vi "读电表参数.vi"(4 "脉冲输入口":u8, 5 "串口号":refnum<visa-resource-name>) -> (1 "应答":string)   [LabVIEW 2014]
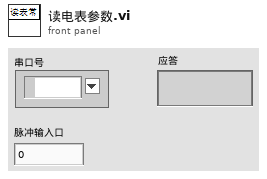
[diagram p1: front panel]
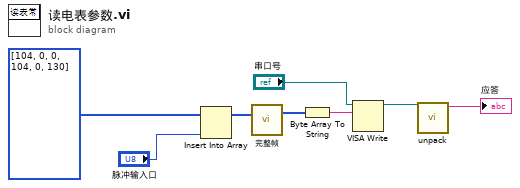
[diagram p0: block diagram]
diagram:
  n1 = Insert Into Array(array=u8[] [104, 0, 0, 104, 0, 130], new element="脉冲输入口") -> (w1:u8[])  [unwired: 1 in]
  n2 = call "完整帧.vi"("不完整帧"=w1) -> ("完整帧"=w2:u8[])  [unwired: 2 in]
  n3 = Byte Array To String(unsigned byte array=w2) -> (string=w3:string)
  n4 = VISA Write(VISA resource name="串口号", write buffer=w3) -> (VISA resource name out=w5:refnum<visa-resource-name>)  [unwired: 1 in, 2 out]
  n5 = call "unpack.vi"("串口号输入"=w5) -> ("应答"=→"应答":string)  [unwired: 5 in, 1 out]
